vi "main.vi"() -> ()   [LabVIEW 2014]
uses:
  <vilib>/Utility/error.llb/DialogType.ctl
panel:
  out "Warning Text":string
  out "Warning":bool
  in  "Temp limits":cluster{"Min (0)":dbl, "Max (25)":dbl}={"Min (0)"=0.0, "Max (25)"=25.0}
  out "Pomiary":dbl[](array[numeric])
  out "Waveform Chart":cluster{"Temp out":dbl, dbl}(graph)
  in  "stop":bool
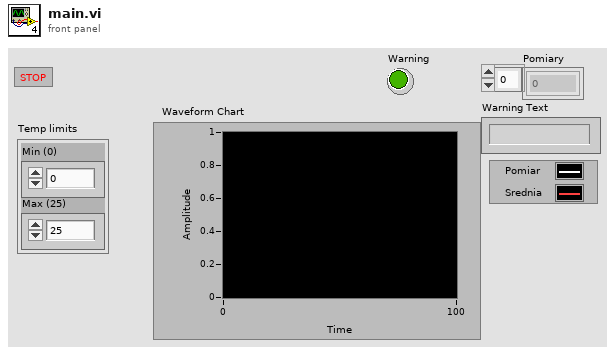
[diagram p1: front panel]
types:
  T1 = typedef "DialogType.ctl" = u16
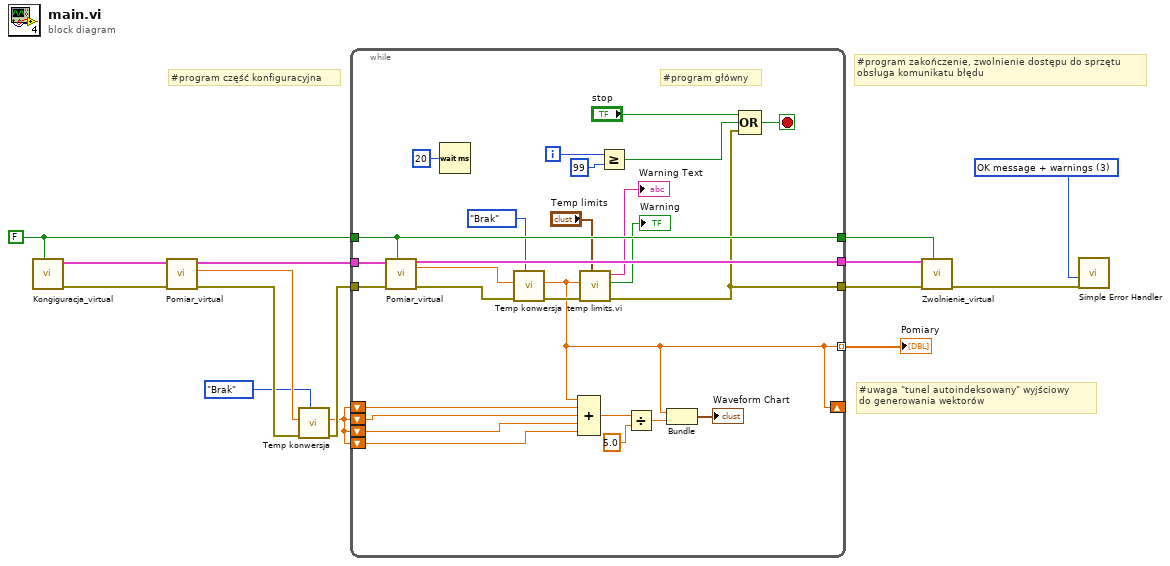
[diagram p0: block diagram]
diagram:
  w10 = T1 3 items=["no dialog", "OK message", "continue or stop message", "OK message + warnings", "continue/stop + warnings"] ("type of dialog (OK msg:1)")
  w15 = FALSE ("Error Generate")
  # "#uwaga \"tunel autoindeksowany\" wyjściowy\ndo generowania wektorów"
  # "#program zakończenie, zwolnienie dostępu do sprzętu\nobsługa komunikatu błędu"
  # "#program część konfiguracyjna"
  n1 = call "Kongiguracja_virtual.vi"("Error Generate"=w15) -> ("error out"=w7:errorcluster, "Reference out"=w6:cluster{"Numeric":dbl, "Boolean":bool})  [unwired: 9 in]
  n2 = call "Pomiar_virtual.vi"("error in (no error)"=w7, "Reference in"=w6) -> ("error out"=w4:errorcluster, "out"=w5:dbl, "Reference out"=w8:cluster{"Numeric":dbl, "Boolean":bool})  [unwired: 7 in]
  n3 = call "Temp konwersja.vi"("Konwersja (stC ->K)"=enum16{"Brak", "stC -> K", "K -> stC"}."Brak", "error in (no error)"=w4, "Temp in (0)"=w5) -> ("error out"=w3:errorcluster, "Temp out"=w1:dbl)  [unwired: 7 in]
  n4 = while {
    tunnel: w3 -> [w42]
    tunnel: w8 -> [w41]
    tunnel: w15 -> [w39]
    tunnel: [w40] -> w14
    tunnel: [w29] -> w13
    tunnel: [w39] -> w12
    tunnel: [w18] -> w9 mode=indexing
    shift-right: [w18] -> _
    shift-left: w1 -> [w24]
    shift-left: w1 -> [w23]
    shift-left: w1 -> [w22]
    shift-left: w1 -> [w21]
    i -> [w36]
    stop <- w37 stop-if-true
    # "#program główny"
    n5 = call "Pomiar_virtual.vi"("Error Generate"=w39, "error in (no error)"=w42, "Reference in"=w41) -> ("error out"=w32:errorcluster, "out"=w33:dbl, "Reference out"=w40:cluster{"Numeric":dbl, "Boolean":bool})  [unwired: 6 in]
    n6 = Wait (ms)(milliseconds to wait=u32 20) -> ()  [unwired: 1 out]
    n7 = call "Temp konwersja.vi"("Konwersja (stC ->K)"=enum16{"Brak", "stC -> K", "K -> stC"}."Brak", "error in (no error)"=w32, "Temp in (0)"=w33) -> ("error out"=w30:errorcluster, "Temp out"=w18:dbl)  [unwired: 7 in]
    n8 = Compound Arithmetic op=ADD(w18, w24, w23, w22, w21) -> (w20:dbl)
    n9 = call "temp limits.vi.vi"("Temp limits"="Temp limits", "error in (no error)"=w30, "TEMP"=w18) -> ("error out"=w29:errorcluster, "Warning"=→"Warning":bool, "Warning Text"=→"Warning Text":string)  [unwired: 6 in]
    n10 = Greater Or Equal?(x=w36, y=99) -> (x >= y?=w34:bool)
    n11 = Divide(x=w20, y=5.0) -> (x/y=w17:dbl)
    n12 = Bundle("Temp out"=w18, w17) -> (→"Waveform Chart":cluster{"Temp out":dbl, dbl})  [unwired: 1 in]
    n13 = Compound Arithmetic op=OR("stop", w34, w29) -> (w37:bool)
  }
  "Pomiary" <- w9
  n14 = call "Zwolnienie_virtual.vi"("Error Generate"=w12, "error in (no error)"=w13, "Reference in"=w14) -> ("error out"=w11:errorcluster)  [unwired: 8 in]
  n15 = call <vilib>:"Simple Error Handler.vi"("type of dialog (OK msg:1)"=w10, "error in (no error)"=w11) -> ()  [unwired: 3 in, 5 out]
